vi "send udp and wait for slow response.vi"(8 "error in":errorcluster, 9 "slow timeout ms (3000)":i32=3000, 10 "command in":string="setwangle>>-0.644700000000", 11 "Device":string) -> (0 "error out":errorcluster, 1 "value for real":string, 2 "error":string, 3 "slow response":string, 5 "No errors":bool)   [LabVIEW 2020]
uses:
  Shared/MySQL/Preset Query Enum.ctl
panel:
  out "no error":bool
  out "correct device?":bool
  out "Slow response device name":string
  out "fast response":string
  out "Port Number":u16
  out "IP Address":string
  in  "Block Slow Port":bool
  out "ID fast":refnum<k16>
  in  "timeout ms (300)":i32=300
  # "setxyzuvw>>1,1,1,1,1,1"
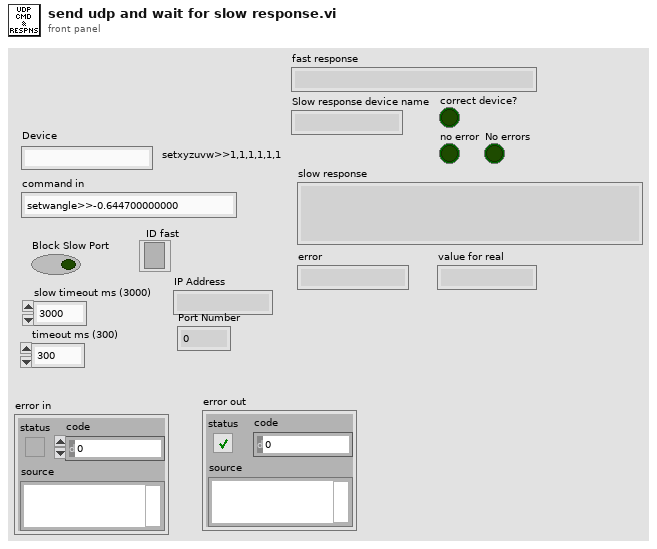
[diagram p1: front panel]
types:
  T1 = typedef "Preset Query Enum.ctl" = enum16{"Get Locations", "Get all IPs and MACs", "Get classes", "Get expt variables to set at scanstart for particular device", "Get expt devices and variables with start values", "Get expt devices and variables (with data to get)", "Get expt devices with data to get", "Get Expt devices and GUIs", "Get all devices basic properties", "Get Virtual Devices Core Info", "Get Expt names", "Get experiment basic properties", "Get experiment alarm variables", "Get MC Ports", "Get device network comm port", "Get devicetype lvclass path", "Get basic device properties", "Get Init Order", "Get all setable variables of a device", "Get device variable aliases", "Get force values of all settable variables", "Get all variables of a devicetype", "Get all variables of a device", "Get plotter details", "Get Saved Scans", "Get Scan Info", "GetGeneralGUIs", "Get expt for plotter", "Get plotter IDs from expt", "Get all devices", "Get all Virtual Devices", "Get all aliases", "Get variable and device info for Virtual Device", "GetItemLocatorIP", "Get IPs for GUIs", "Get DeviceType from Device", "GetLocalPortRange", "GetDevicePresetVariables", "Get Device Configuration", "GetAllPresetNames", "GetAllConfigurationNames", "GetPresetDeviceNames", "GetDeviceAliases", "GetDevicesOfClass"}
  T2 = cluster{"data[0]":string, "data[1]":string, "data[2]":string, "data[3]":string, "data[4]":string, "data[5]":string, "data[6]":string, "data[7]":string, "data[8]":string}
  T3 = cluster{"data[0]":string, "data[1]":string, "data[2]":string, "data[3]":string, "data[4]":string, "data[5]":string, "data[6]":string, "data[7]":string, "data[8]":string}[]
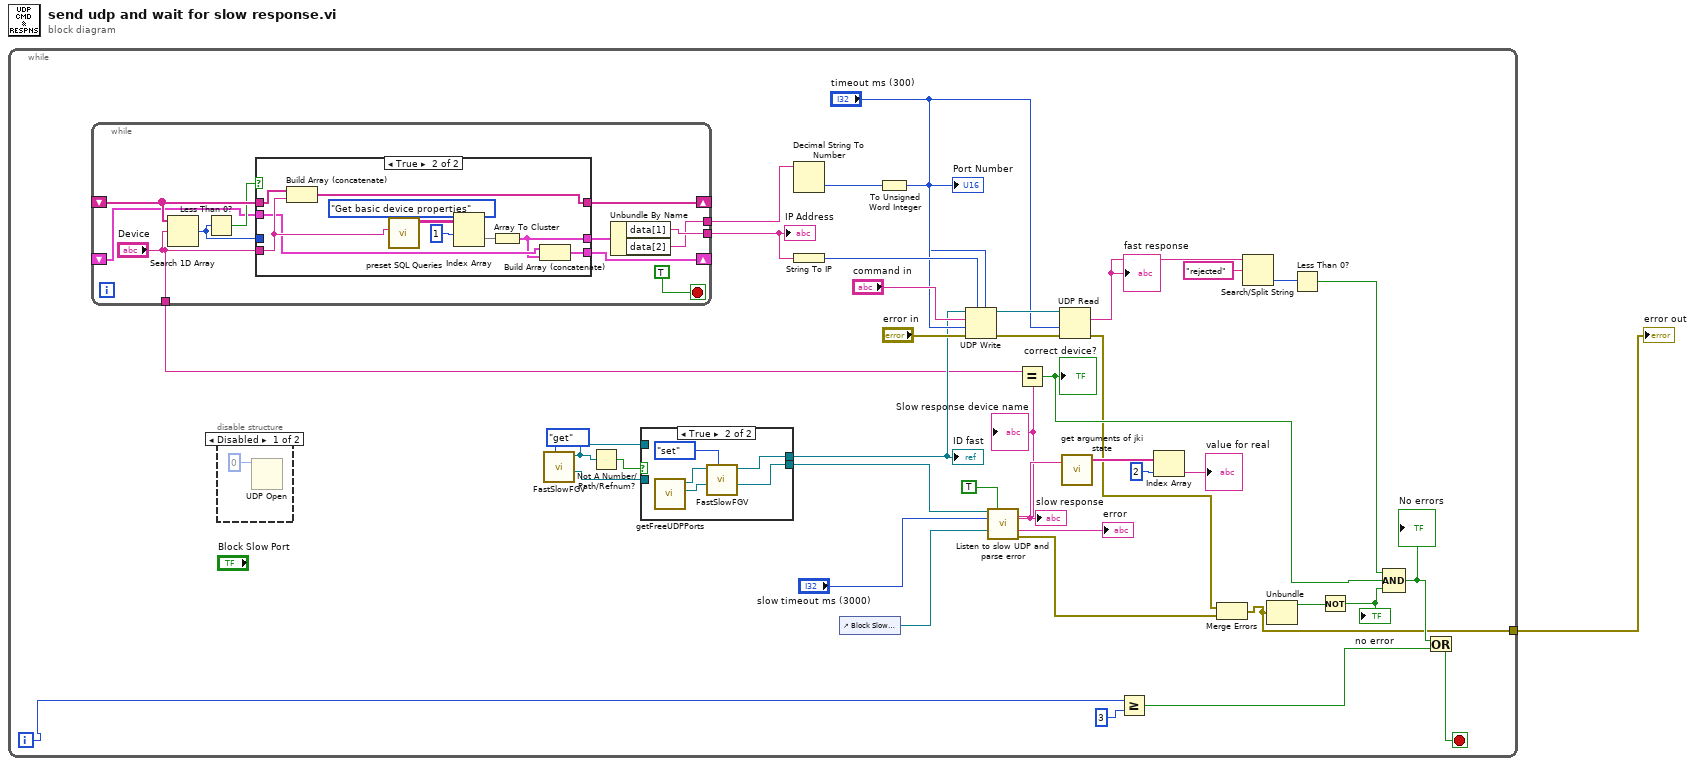
[diagram p0: block diagram]
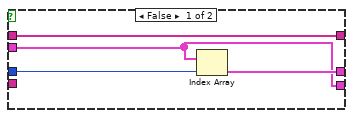
[diagram p3: hidden frame]
diagram:
  n1 = while {
    tunnel: [w2] -> w1
    i -> [w17]
    stop <- w13 stop-if-true
    n2 = while {
      shift-right: [w56] -> _
      shift-left: _ -> [w55]
      tunnel: [w58] -> w24
      tunnel: [w57] -> w23
      shift-right: [w52] -> _
      shift-left: _ -> [w53]
      tunnel: ["Device"] -> w12
      stop <- TRUE stop-if-true
      n3 = Search 1D Array(1D array=w55, element="Device") -> (index of element=w51:i32)  [unwired: 1 in]
      n4 = Less Than 0?(x=w51) -> (x < 0?=w54:bool)
      n5 = case shown="True" w54 {
        tunnel: [w62 w66] -> w59
        tunnel: [w64 w70] -> w56
        tunnel: w55 -> [w64 w69]
        tunnel: "Device" -> [_ w68]
        tunnel: w53 -> [w61 w67]
        tunnel: [w61 w65] -> w52
        tunnel: w51 -> [w63 _]
        frame False {
          n6 = Index Array(array=w61, index=w63) -> (element=w62:T2)
        }
        frame True {
          n7 = Build Array (concatenate)(w69, w68) -> (w70:string[])
          n8 = call "preset SQL Queries.vi"("Device/Devicetype name\n/Plotter.id/ScanName#"=w68, "Preset Query"=Preset_Query_Enum."Get basic device properties") -> ("data"=w73:string[][])  [unwired: 7 in, 2 out]
          n9 = Index Array(array=w73, index (row)=1) -> (element=w74:string[])  [unwired: 1 in]
          n10 = Array To Cluster(array=w74) -> (cluster=w66:T2)
          n11 = Build Array (concatenate)(w67, w66) -> (w65:T3)
        }
      }
      n12 = Unbundle By Name(w59) -> ("data[1]"=w58:string, "data[2]"=w57:string)
    }
    "IP Address" <- w24
    n13 = disable-structure shown="Disabled" {
      frame Disabled {
        n14 = UDP Open(11:u16 0 ("port")) -> ()  [unwired: 4 in, 3 out]
      }
      frame Enabled {
      }
    }
    n15 = call "FastSlowFGV.vi"("Command"=enum16{"get", "set", "init"}."get") -> ("slow ID out"=w19:refnum<k16>, "fast ID out"=w20:refnum<k16>)  [unwired: 9 in]
    n16 = Not A Number/Path/Refnum?(number/path/refnum=w20) -> (NaN/Path/Refnum?=w21:bool)
    n17 = case shown="True" w21 {
      tunnel: [w43 w47] -> w36
      tunnel: [w44 w48] -> w29
      tunnel: w20 -> [w44 _]
      tunnel: w19 -> [w43 _]
      frame False {
      }
      frame True {
        n18 = call "getFreeUDPPorts.vi"() -> ("slow"=w45:refnum<k16>, "fast"=w46:refnum<k16>)  [unwired: 8 in, 2 out]
        n19 = call "FastSlowFGV.vi"("Command"=enum16{"get", "set", "init"}."set", "slow ID"=w45, "fast ID"=w46) -> ("slow ID out"=w47:refnum<k16>, "fast ID out"=w48:refnum<k16>)  [unwired: 7 in]
      }
    }
    "ID fast" <- w29
    n20 = Decimal String To Number(string=w23) -> (number=w32:i32)  [unwired: 2 in, 1 out]
    n21 = String To IP(1:w24) -> (0:w39:u32)
    n22 = control-ref of="Block Slow Port"() -> (w30:refnum<vi>)
    n23 = To Unsigned Word Integer(number=w32) -> (unsigned 16bit integer=w31:u16)
    "Port Number" <- w31
    n24 = UDP Write(address=w39, port or service name=w31, connection ID=w29, data in="command in", 8:"error in", 9:"timeout ms (300)") -> (error out=w38:errorcluster, 3:w40:refnum<k16>)
    n25 = call "Listen to slow UDP and parse error.vi"("ID slow"=w36, "command accepted"=TRUE, "timeout ms (25000)"="slow timeout ms (3000)", "block slow port 2"=w30) -> ("Whatami"=w11:string, "data out"=w28:string, "value"=→"error":string, "error out"=w15:errorcluster)  [unwired: 4 in, 4 out]
    "slow response" <- w28
    "Slow response device name" <- w11
    n26 = Equal?(x=w12, y=w11) -> (x = y?=w10:bool)
    "correct device?" <- w10
    n27 = UDP Read(connection ID=w40, timeout ms (25000)="timeout ms (300)", 8:w38) -> (data out=w7:string, error out=w3:errorcluster)  [unwired: 1 in, 3 out]
    "fast response" <- w7
    n28 = call "get arguments of jki state.vi"("jki arguments"=w28) -> ("Argument Array"=w27:string[])  [unwired: 1 in, 2 out]
    n29 = Greater Or Equal?(x=w17, y=3 ("x")) -> (x >= y?=w14:bool)
    n30 = Index Array(array=w27, index=2) -> (element=→"value for real":string)
    n31 = Merge Errors(w3, w15) -> (w2:errorcluster)
    n32 = Search/Split String(string=w7, search string/char (-)="rejected") -> (offset of match=w5:i32)  [unwired: 1 in, 2 out]
    n33 = Unbundle(w2) -> ("status"=w18:bool)  [unwired: 2 out]
    n34 = Less Than 0?(x=w5) -> (x < 0?=w4:bool)
    n35 = Not(x=w18) -> (.not. x?=w9:bool)
    "no error" <- w9
    n36 = Compound Arithmetic op=AND(w4, w10, w9) -> (w8:bool)
    "No errors" <- w8
    n37 = Or(x=w8, y=w14) -> (x .or. y?=w13:bool)
  }
  "error out" <- w1
